vi "Agilent 34420 Read Multiple.vi"() -> ()   [LabVIEW 2021]
doc: "This example shows how to configure a simple measurement and take multiple readings."
uses:
  <instrlib>/Agilent 34420/Public/Data/Read (Multiple Points).vi
  <instrlib>/Agilent 34420/Agilent 34420.lvlib
panel:
  in  "Maximum Time (30000 ms)":u32=30000
  in  "Function (0: DC Volts)":u16(ring) items=["DC Volts", "DC Voltage Ratio", "DC Voltage Difference", "2 Wire Resistance", "4 Wire Resistance", "Temperature"]
  in  "Serial Configuration":T1={"Baud Rate"=9600, "Parity"=0, "Data Bits"=8} {"Data Bits" items=["7"=7, "8"=8]; "Parity" items=["None", "Odd", "Even", "Mark", "Space"]; "Baud Rate" items=["300"=300, "600"=600, "1200"=1200, "2400"=2400, "4800"=4800, "9600"=9600]}
  out "Measurements":dbl[](array[numeric])
  in  "Sample Count (25)":i32=25
  in  "VISA resource name":refnum<visa-resource-name>
  # "(c) 2008-2015 National Instruments Corp.  ALL RIGHTS RESERVED."
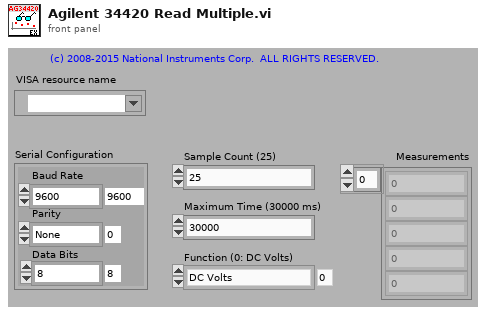
[diagram p1: front panel]
types:
  T1 = cluster{"Baud Rate":u32, "Parity":u16, "Data Bits":u16}
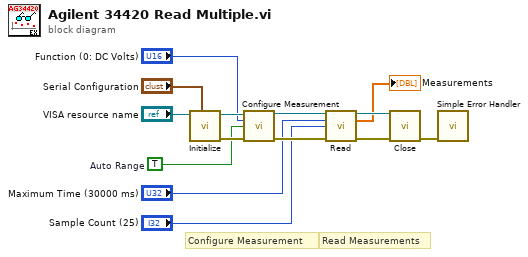
[diagram p0: block diagram]
diagram:
  w10 = TRUE  # Auto Range
  # "Read Measurements"
  # "Configure Measurement"
  n1 = call <instrlib>:"Initialize.vi"("Serial Configuration"="Serial Configuration", "VISA resource name"="VISA resource name") -> ("error out"=w11:errorcluster, "VISA resource name out"=w12:refnum<visa-resource-name>)  [unwired: 8 in]
  n2 = call <instrlib>:"Configure Measurement.vi"("VISA resource name"=w12, "Function (0: DC Volts)"="Function (0: DC Volts)", "Auto Range (T:Enable)"=w10, "error in (no error)"=w11) -> ("VISA resource name out"=w7:refnum<visa-resource-name>, "error out"=w8:errorcluster)  [unwired: 10 in]
  n3 = call-poly <instrlib>:"Read.vi"("VISA resource name"=w7, "Maximum Time (30000 ms)"="Maximum Time (30000 ms)", "Sample Count (1)"="Sample Count (25)", "error in (no error)"=w8) -> ("VISA resource name out"=w6:refnum<visa-resource-name>, "Measurements"=→"Measurements":dbl[], "error out"=w9:errorcluster)  [unwired: 9 in]
  n4 = call <instrlib>:"Close.vi"("error in (no error)"=w9, "VISA resource name"=w6) -> ("error out"=w14:errorcluster)  [unwired: 9 in]
  n5 = call <vilib>:"Simple Error Handler.vi"("error in (no error)"=w14) -> ()  [unwired: 4 in, 5 out]
